vi "Reset.vi"(8 "error in (no error)":errorcluster caption="错误输入（无错误）", 11 "Enumerator 输入":refnum<class "Enumerator.lvclass"> caption="DNL_LabVIEW Object in") -> (0 "error out":errorcluster caption="错误输出", 3 "Enumerator 输出":refnum<class "Enumerator.lvclass"> caption="DNL_LabVIEW Object out")   [LabVIEW 2012, in "Enumerator.lvclass"]
uses:
  Enumerator.lvclass
  Enumerator.lvclass/Enumerator.ctl
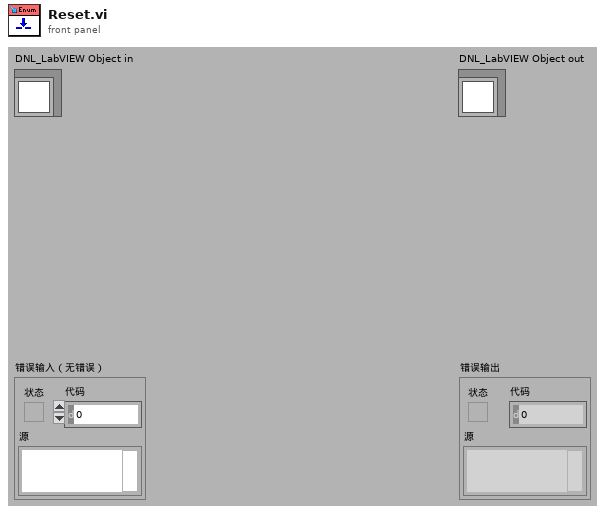
[diagram p1: front panel]
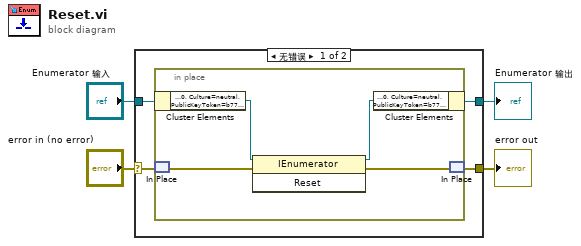
[diagram p0: block diagram]
diagram:
  n1 = case shown="无错误" "error in (no error)" {
    selector: "error in (no error)" -> [w7 w14]
    tunnel: [w6 w14] -> w3
    tunnel: [w5 w13] -> w1
    tunnel: "Enumerator 输入" -> [w8 w13]
    frame No Error {
      n2 = in-place {
        n3 = in-place-cluster #1(w8) -> ("Enumerator"=w12:refnum<k24>)
        n4 = in-place-match #2(w7) -> (w11:errorcluster)
        n5 = invoke class="IEnumerator" method="Reset"(reference=w12, error in=w11) -> (reference out=w9:refnum<k24>, error out=w10:errorcluster)  [unwired: 1 in, 1 out]
        n6 = in-place-cluster #1("Enumerator"=w9) -> (w5:refnum<class "Enumerator.lvclass">)
        n7 = in-place-match #2(w10) -> (w6:errorcluster)
      }
    }
    frame Error {
    }
  }
  "error out" <- w3
  "Enumerator 输出" <- w1
